vi "FGV Driver Data.vi"(5 "DUT channel (1-11)":i32=1, 6 "Mode":T2, 7 "DUT index(1-60)":i32, 8 "error in (no error)":errorcluster, 9 "FGV enum(Read)":T3=enum."Read", 11 "data":variant) -> (0 "error out":errorcluster, 1 "Short Circuits?":bool[](array[boolean]), 2 "DUT SC":bool, 3 "60 DRV data":T1[](array[typedef]))   [LabVIEW 2018, in "Application.lvlib"]
uses:
  Application.lvlib
  FGV DRV data.ctl
  DUT data Mode.ctl
  DRV cluster 2.ctl
  eMICs Cluster.ctl
  eMIC response.ctl
panel:
  out "Processed Data":T1[](array[typedef])
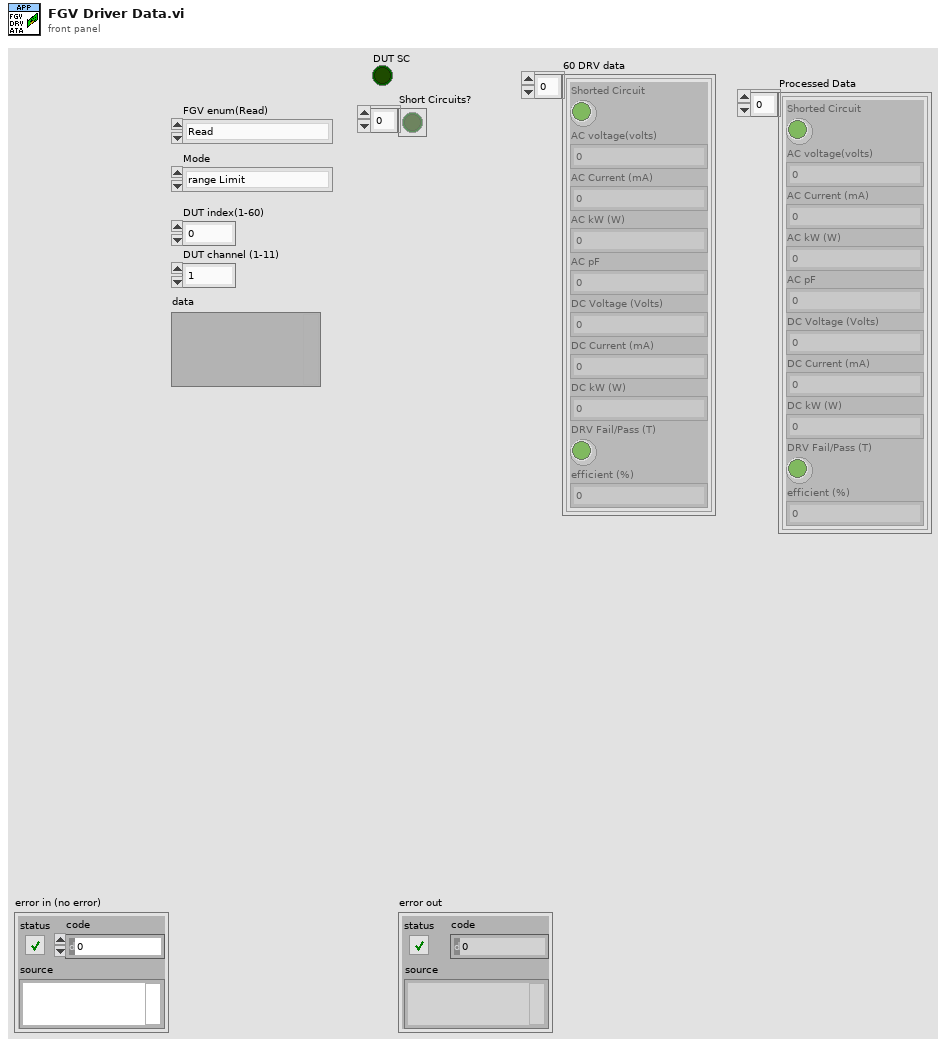
[diagram p1: front panel]
types:
  T1 = typedef "Application.lvlib/DRV cluster 2.ctl" = cluster{"Shorted Circuit":bool, "AC voltage(volts)":dbl, "AC Current (mA)":dbl, "AC kW (W)":dbl, "AC pF ":dbl, "DC Voltage (Volts)":dbl, "DC Current (mA)":dbl, "DC kW (W)":dbl, "DRV Fail/Pass (T)":bool, "efficient (%)":dbl}
  T2 = typedef "Application.lvlib/DUT data Mode.ctl" = enum16{"range Limit", "Short Circuits", "AC parameter", "AC parameter 1", "DC parameter"}
  T3 = typedef "Application.lvlib/FGV DRV data.ctl" = enum16{"Init", "Write", "Read", "Process"}
  T4 = typedef "Application.lvlib/eMICs Cluster.ctl" = cluster{"eMIC 1":T5, "eMIC 2":T5, "eMIC 3":T5, "eMIC 4":T5, "eMIC 5":T5, "eMIC 6":T5}
  T5 = typedef "Application.lvlib/eMIC response.ctl" = cluster{"ACV":dbl, "ACI":dbl, "pF":dbl, "kW":dbl, "Freq":dbl, "kvar":dbl}
  T6 = typedef "Application.lvlib/DRV stand.ctl" = cluster{"SAP ID":string, "Name":string, "AC characteristics":cluster{"Voltage":cluster{"Min":dbl, "Max":dbl}, "Current":cluster{"Min":dbl, "Max":dbl}, "kW":cluster{"Min":dbl, "Max":dbl}, "PF":cluster{"Min":dbl, "Max":dbl}}, "DC characteristics":cluster{"Voltage":cluster{"Min":dbl, "Max":dbl}, "Current":cluster{"Min":dbl, "Max":dbl}, "Effect":cluster{"Min":dbl, "Max":dbl}}, "Sub-Test":cluster{"ACV":bool, "ACI":bool, "kW":bool, "PF":bool, "DCV":bool, "DCI":bool, "efficiency":bool}}
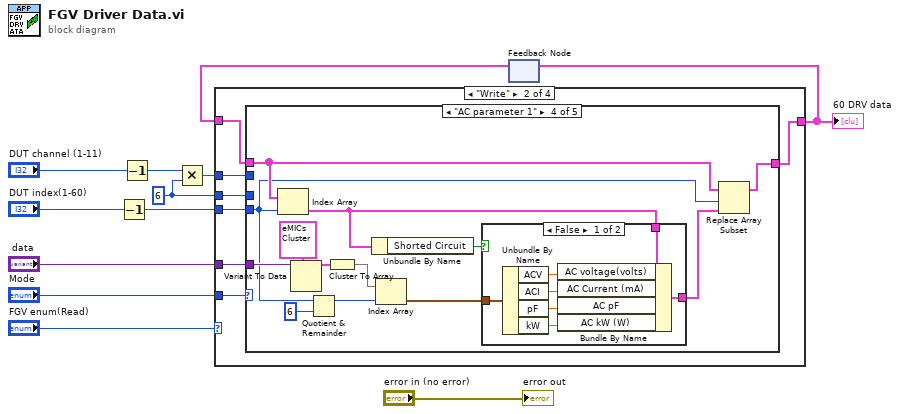
[diagram p0: block diagram]
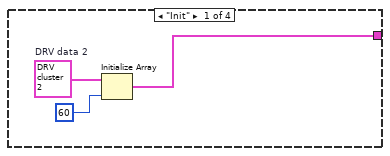
[diagram p2: hidden frame]
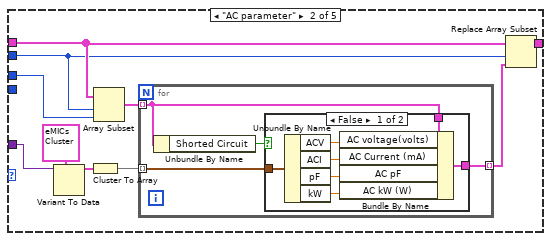
[diagram p4: hidden frame]
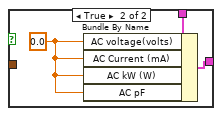
[diagram p5: hidden frame]
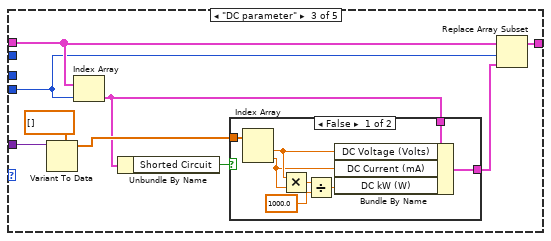
[diagram p6: hidden frame]
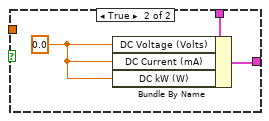
[diagram p7: hidden frame]
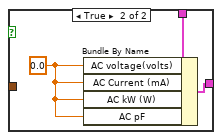
[diagram p8: hidden frame]
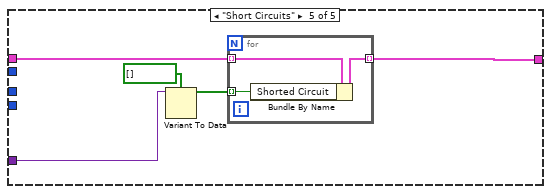
[diagram p9: hidden frame]
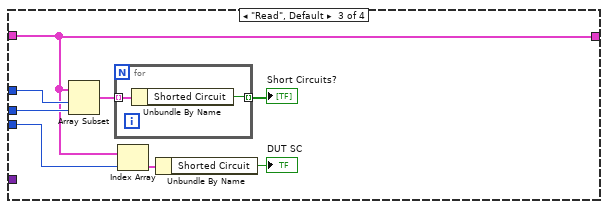
[diagram p10: hidden frame]
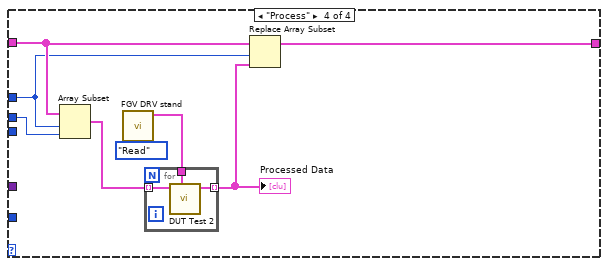
[diagram p11: hidden frame]
diagram:
  w4 = 6 ("length")
  n1 = Decrement(x="DUT index(1-60)") -> (x-1=w1:i32)
  n2 = Decrement(x="DUT channel (1-11)") -> (x-1=w6:i32)
  n3 = Multiply(x=w6, y=w4) -> (x*y=w5:i32)
  n4 = feedback #1() -> (w11:T1[])  [unwired: 1 in]
  n5 = case shown="\"Write\"" "FGV enum(Read)" {
    tunnel: [w14 w20 w102 w114] -> w3
    tunnel: w11 -> [_ w21 w102 w116]
    tunnel: "Mode" -> [_ w22 _ _]
    tunnel: "data" -> [_ w19 _ _]
    tunnel: w5 -> [_ w18 w106 w113]
    tunnel: w4 -> [_ w17 w105 w109]
    tunnel: w1 -> [_ w16 w101 _]
    frame "Init" {
      w13 = T1 {"Shorted Circuit"=TRUE, "AC voltage(volts)"=0.0, "AC Current (mA)"=0.0, "AC kW (W)"=0.0, "AC pF "=0.0, "DC Voltage (Volts)"=0.0, "DC Current (mA)"=0.0, "DC kW (W)"=0.0, "DRV Fail/Pass (T)"=TRUE, "efficient (%)"=0.0}  # DRV data 2
      n6 = Initialize Array(w13, 60 ("dimension size")) -> (w14:T1[])
    }
    frame "Write" {
      n7 = case shown="\"AC parameter 1\"" w22 {
        tunnel: w21 -> [w23 w30 w56 w80 w95]
        tunnel: [w23 w31 w55 w79 w94] -> w20
        tunnel: w19 -> [_ w27 w53 w74 w93]
        tunnel: w18 -> [_ w29 _ _ _]
        tunnel: w17 -> [_ w28 _ _ _]
        tunnel: w16 -> [_ _ w48 w72 _]
        frame "range Limit", Default {
        }
        frame "AC parameter" {
          n8 = Variant To Data(type=T4 {"eMIC 1"={"ACV"=0.0, "ACI"=0.0, "pF"=0.0, "kW"=0.0, "Freq"=0.0, "kvar"=0.0}, "eMIC 2"={"ACV"=0.0, "ACI"=0.0, "pF"=0.0, "kW"=0.0, "Freq"=0.0, "kvar"=0.0}, "eMIC 3"={"ACV"=0.0, "ACI"=0.0, "pF"=0.0, "kW"=0.0, "Freq"=0.0, "kvar"=0.0}, "eMIC 4"={"ACV"=0.0, "ACI"=0.0, "pF"=0.0, "kW"=0.0, "Freq"=0.0, "kvar"=0.0}, "eMIC 5"={"ACV"=0.0, "ACI"=0.0, "pF"=0.0, "kW"=0.0, "Freq"=0.0, "kvar"=0.0}, "eMIC 6"={"ACV"=0.0, "ACI"=0.0, "pF"=0.0, "kW"=0.0, "Freq"=0.0, "kvar"=0.0}} ("eMICs cluster"), Variant=w27) -> (data=w25:T4)  [unwired: 1 in, 1 out]
          n9 = Cluster To Array(cluster=w25) -> (array=w24:T5[])
          n10 = Array Subset(array=w30, index=w29, length=w28) -> (w33:T1[])
          n11 = for {
            tunnel: w33 -> [w36] mode=indexing
            tunnel: w24 -> [w34] mode=indexing
            tunnel: [w37] -> w32 mode=indexing
            n12 = Unbundle By Name(w36) -> ("Shorted Circuit"=w35:bool)
            n13 = case shown="False" w35 {
              tunnel: w34 -> [w44 _]
              tunnel: [w43 w46] -> w37
              tunnel: w36 -> [w38 w47]
              frame False {
                n14 = Unbundle By Name(w44) -> ("ACV"=w42:dbl, "ACI"=w41:dbl, "pF"=w40:dbl, "kW"=w39:dbl)
                n15 = Bundle By Name(cluster=w38, "AC voltage(volts)"=w42, "AC Current (mA)"=w41, "AC pF"=w40, "AC kW (W)"=w39) -> (w43:T1)
              }
              frame True {
                w45 = 0.0 ("AC voltage(volts)")
                n16 = Bundle By Name(cluster=w47, "AC voltage(volts)"=w45, "AC Current (mA)"=w45, "AC kW (W)"=w45, "AC pF"=w45) -> (w46:T1)
              }
            }
          }
          n17 = Replace Array Subset(array=w30, new element=w32, index=w29) -> (w31:T1[])
        }
        frame "DC parameter" {
          n18 = Variant To Data(type=dbl[] [], Variant=w53) -> (data=w52:dbl[])  [unwired: 1 in, 1 out]
          n19 = Index Array(array=w56, index=w48) -> (element=w50:T1)
          n20 = Unbundle By Name(w50) -> ("Shorted Circuit"=w49:bool)
          n21 = case shown="False" w49 {
            tunnel: w52 -> [w64 _]
            tunnel: [w58 w66] -> w51
            tunnel: w50 -> [w57 w67]
            frame False {
              n22 = Index Array(array=w64) -> (element #1=w63:dbl, element #2=w62:dbl)  [unwired: 2 in]
              n23 = Multiply(x=w63, y=w62) -> (x*y=w61:dbl)
              n24 = Divide(x=w61, y=1000.0) -> (x/y=w59:dbl)
              n25 = Bundle By Name(cluster=w57, "DC Voltage (Volts)"=w63, "DC Current (mA)"=w62, "DC kW (W)"=w59) -> (w58:T1)
            }
            frame True {
              w65 = 0.0 ("DC Voltage (Volts)")
              n26 = Bundle By Name(cluster=w67, "DC Voltage (Volts)"=w65, "DC Current (mA)"=w65, "DC kW (W)"=w65) -> (w66:T1)
            }
          }
          n27 = Replace Array Subset(array=w56, new element=w51, index=w48) -> (w55:T1[])
        }
        frame "AC parameter 1" {
          n28 = Index Array(array=w80, index=w72) -> (element=w77:T1)
          n29 = Variant To Data(type=T4 {"eMIC 1"={"ACV"=0.0, "ACI"=0.0, "pF"=0.0, "kW"=0.0, "Freq"=0.0, "kvar"=0.0}, "eMIC 2"={"ACV"=0.0, "ACI"=0.0, "pF"=0.0, "kW"=0.0, "Freq"=0.0, "kvar"=0.0}, "eMIC 3"={"ACV"=0.0, "ACI"=0.0, "pF"=0.0, "kW"=0.0, "Freq"=0.0, "kvar"=0.0}, "eMIC 4"={"ACV"=0.0, "ACI"=0.0, "pF"=0.0, "kW"=0.0, "Freq"=0.0, "kvar"=0.0}, "eMIC 5"={"ACV"=0.0, "ACI"=0.0, "pF"=0.0, "kW"=0.0, "Freq"=0.0, "kvar"=0.0}, "eMIC 6"={"ACV"=0.0, "ACI"=0.0, "pF"=0.0, "kW"=0.0, "Freq"=0.0, "kvar"=0.0}} ("eMICs cluster"), Variant=w74) -> (data=w75:T4)  [unwired: 1 in, 1 out]
          n30 = Quotient & Remainder(x=w72, y=6) -> (x-y*floor(x/y)=w70:i32)  [unwired: 1 out]
          n31 = Cluster To Array(cluster=w75) -> (array=w73:T5[])
          n32 = Unbundle By Name(w77) -> ("Shorted Circuit"=w78:bool)
          n33 = Index Array(array=w73, index=w70) -> (element=w68:T5)
          n34 = case shown="False" w78 {
            tunnel: w68 -> [w87 _]
            tunnel: [w86 w89] -> w69
            tunnel: w77 -> [w81 w90]
            frame False {
              n35 = Unbundle By Name(w87) -> ("ACV"=w85:dbl, "ACI"=w84:dbl, "pF"=w83:dbl, "kW"=w82:dbl)
              n36 = Bundle By Name(cluster=w81, "AC voltage(volts)"=w85, "AC Current (mA)"=w84, "AC pF"=w83, "AC kW (W)"=w82) -> (w86:T1)
            }
            frame True {
              w88 = 0.0 ("AC voltage(volts)")
              n37 = Bundle By Name(cluster=w90, "AC voltage(volts)"=w88, "AC Current (mA)"=w88, "AC kW (W)"=w88, "AC pF"=w88) -> (w89:T1)
            }
          }
          n38 = Replace Array Subset(array=w80, new element=w69, index=w72) -> (w79:T1[])
        }
        frame "Short Circuits" {
          n39 = Variant To Data(type=bool[] [], Variant=w93) -> (data=w91:bool[])  [unwired: 1 in, 1 out]
          n40 = for {
            tunnel: w95 -> [w98] mode=indexing
            tunnel: [w97] -> w94 mode=indexing
            tunnel: w91 -> [w96] mode=indexing
            n41 = Bundle By Name(cluster=w98, "Shorted Circuit"=w96) -> (w97:T1)
          }
        }
      }
    }
    frame "Read", Default {
      n42 = Array Subset(array=w102, index=w106, length=w105) -> (w104:T1[])
      n43 = for {
        tunnel: w104 -> [w108] mode=indexing
        tunnel: [w107] -> w103 mode=indexing
        n44 = Unbundle By Name(w108) -> ("Shorted Circuit"=w107:bool)
      }
      "Short Circuits?" <- w103
      n45 = Index Array(array=w102, index=w101) -> (element=w100:T1)
      n46 = Unbundle By Name(w100) -> ("Shorted Circuit"=→"DUT SC":bool)
    }
    frame "Process" {
      n47 = Array Subset(array=w116, index=w113, length=w109) -> (w115:T1[])
      n48 = call "FGV DRV stand.vi"("Enum"=enum16{"Write", "Read"}."Read") -> ("DRV stand out"=w110:T6)  [unwired: 10 in]
      n49 = for {
        tunnel: w115 -> [w119] mode=indexing
        tunnel: [w118] -> w112 mode=indexing
        tunnel: w110 -> [w117]
        n50 = call "DUT Test 2.vi"("DRV stand"=w117, "DRV data"=w119) -> ("DRV data 2"=w118:T1)  [unwired: 6 in, 3 out]
      }
      "Processed Data" <- w112
      n51 = Replace Array Subset(array=w116, new element=w112, index=w113) -> (w114:T1[])
    }
  }
  "60 DRV data" <- w3
  n52 = feedback-in #1(w3) -> ()
  "error out" <- "error in (no error)"
